vi "Read Read Only.vi"(8 "error in (no error)":errorcluster, 11 "Const_CPLX_DBL in":refnum<class "Const_CPLX_DBL.lvclass">) -> (0 "error out":errorcluster, 2 "Read Only":bool, 3 "Const_CPLX_DBL out":refnum<class "Const_CPLX_DBL.lvclass">)   [LabVIEW 2021, in "Const_CPLX_DBL.lvclass"]
uses:
  Const_CPLX_DBL.lvclass
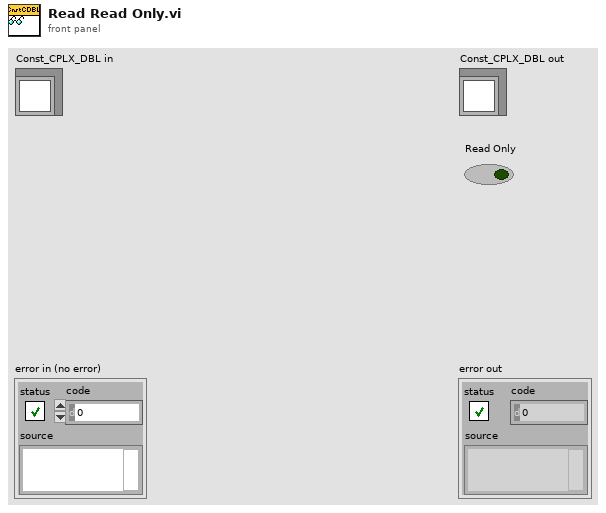
[diagram p1: front panel]
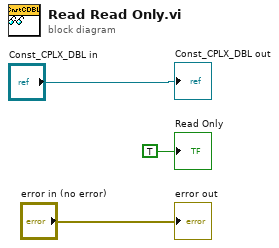
[diagram p0: block diagram]
diagram:
  "error out" <- "error in (no error)"
  "Const_CPLX_DBL out" <- "Const_CPLX_DBL in"
  "Read Only" <- TRUE ("Read Only")
